vi "Software Update HCC Filter Desired File Paths.vi"(8 "Error In":errorcluster, 9 "Update Files (Option 1-24)":i32[](array[numeric]), 10 "Index of File Path":i32[](array[numeric]), 11 "All File Paths":path[](array[path])) -> (0 "Error Out":errorcluster, 3 "Desired File Paths":path[](array[path]))   [LabVIEW 2016]
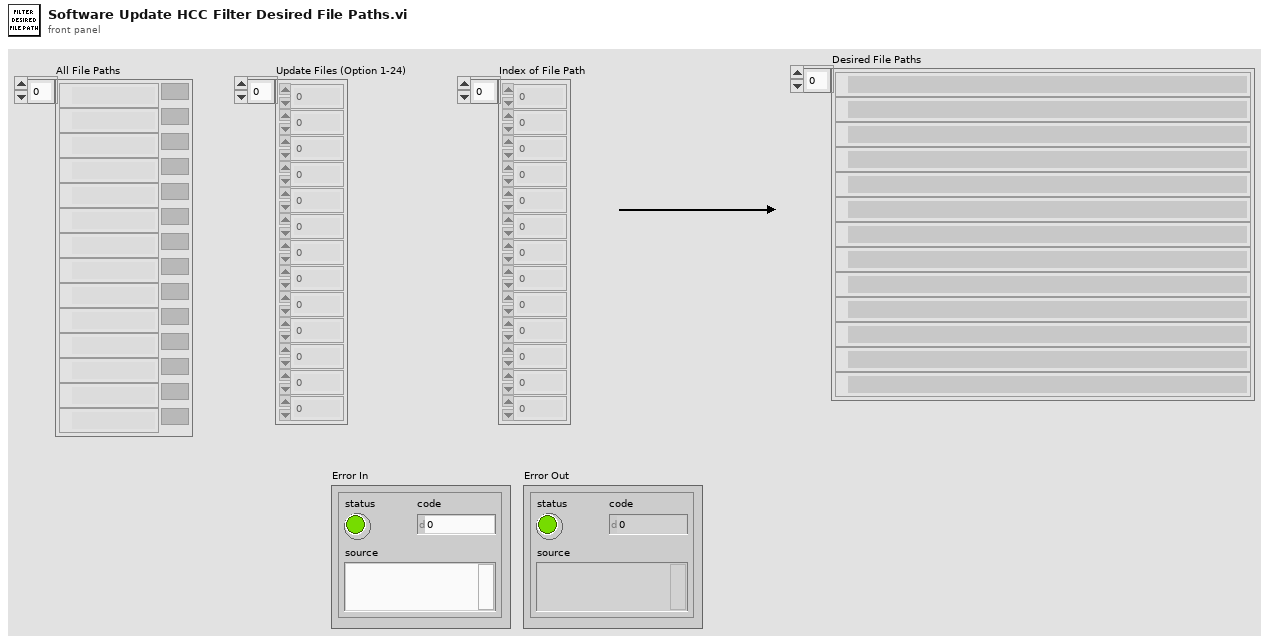
[diagram p1: front panel]
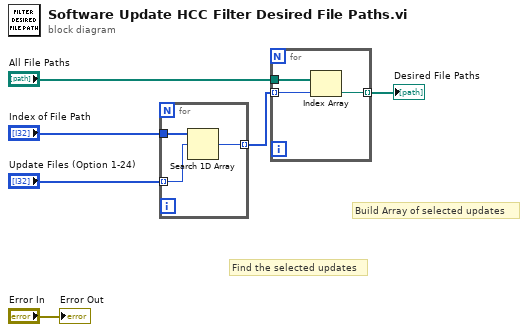
[diagram p0: block diagram]
diagram:
  # "Find the selected updates"
  # "Build Array of selected updates"
  n1 = for {
    tunnel: "Update Files (Option 1-24)" -> [w7] mode=indexing
    tunnel: "Index of File Path" -> [w8]
    tunnel: [w9] -> w4 mode=indexing
    n2 = Search 1D Array(1D array=w8, element=w7) -> (index of element=w9:i32)  [unwired: 1 in]
  }
  n3 = for {
    tunnel: "All File Paths" -> [w12]
    tunnel: w4 -> [w11] mode=indexing
    tunnel: [w10] -> w2 mode=indexing
    n4 = Index Array(array=w12, index=w11) -> (element=w10:path)
  }
  "Desired File Paths" <- w2
  "Error Out" <- "Error In"
